vi "Server.vi"() -> ()   [LabVIEW 2020]
uses:
  source/Value/Value/Value.lvclass
  source/Server/Server/Server.lvclass
  source/Server/Source/Source.lvclass
  source/Server/Server.lvlib
  2ff34015-19c1-41a1-a1e8-1eab219b517a.vi
  7054ff5f-c778-4b9f-bf9e-4a55a1cdcc59.vi
  4fabb87d-4e15-4188-883f-208453235fd8.vi
  6c06fff3-e822-4e92-b24f-bdc271668697.vi
  0073a8bc-0586-4490-b945-e374f2b6411c.vi
panel:
  in  "Value":dbl
  in  "Increment":bool
  in  "stop":bool
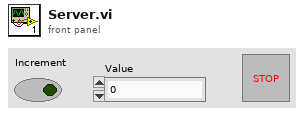
[diagram p1: front panel]
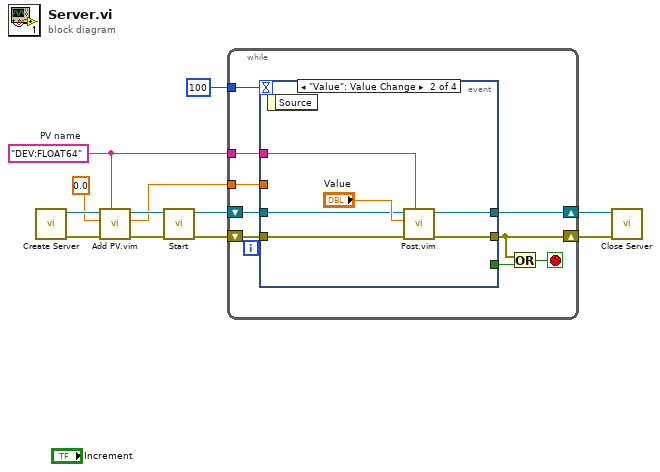
[diagram p0: block diagram]
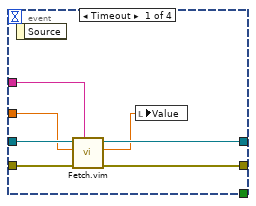
[diagram p2: hidden frame]
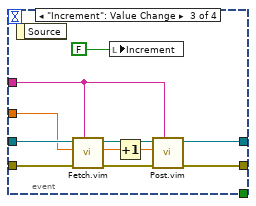
[diagram p3: hidden frame]
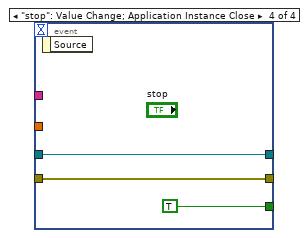
[diagram p4: hidden frame]
diagram:
  w4 = "DEV:FLOAT64"  # PV name
  n1 = call "Create Server.vi"() -> ("error out"=w12:errorcluster, "Server"=w11:refnum<class "Server.lvclass">)  [unwired: 10 in]
  n2 = call "Add PV.vim"("PV name"=w4, "error in"=w12, "initial value"=0.0, "Server in"=w11) -> ("error out"=w7:errorcluster, "value"=w1:dbl, "Server out"=w8:refnum<class "Server.lvclass">)  [unwired: 5 in]
  n3 = call-dynamic "Start.vi"("error in (no error)"=w7, "Server in"=w8) -> ("error out"=w5:errorcluster, "Server out"=w6:refnum<class "Server.lvclass">)  [unwired: 8 in]
  n4 = while {
    tunnel: w4 -> [w20]
    shift-right: [w18] -> w9
    shift-left: w6 -> [w19]
    shift-right: [w15] -> w10
    shift-left: w5 -> [w21]
    tunnel: 100 ("Numeric") -> [w14]
    tunnel: w1 -> [w13]
    stop <- w16 stop-if-true
    n5 = event shown="[1] \"Value\": Value Change" {
      selector: _ -> [_ _ _ _]
      dyn-events: _ -> [_ _ _ _]
      timeout: w14 -> [_ _ _ _]
      tunnel: w21 -> [w27 w34 w45 w47]
      tunnel: w20 -> [w28 w32 w37 _]
      tunnel: w19 -> [w26 w31 w44 w46]
      tunnel: [w24 w29 w35 w47] -> w15
      tunnel: [w25 w30 w36 w46] -> w18
      tunnel: [_ _ _ TRUE] -> w17
      tunnel: w13 -> [w23 _ w41 _]
      event Timeout {
        n6 = event-data() -> ()  [unwired: 1 in, 1 out]
        n7 = call "Fetch.vim"("PV name"=w28, "error in"=w27, "default"=w23, "Server in"=w26) -> ("error out"=w24:errorcluster, "value"=w22:dbl, "Server out"=w25:refnum<class "Server.lvclass">)  [unwired: 5 in]
        n8 = local write "Value"(w22) -> ()
      }
      event "Value": Value Change {
        n9 = event-data() -> ()  [unwired: 1 in, 1 out]
        n10 = call "Post.vim"("PV name"=w32, "error in"=w34, "value in"="Value", "Server in"=w31) -> ("error out"=w29:errorcluster, "Server out"=w30:refnum<class "Server.lvclass">)  [unwired: 5 in, 1 out]
      }
      event "Increment": Value Change {
        n11 = event-data() -> ()  [unwired: 1 in, 1 out]
        n12 = call "Fetch.vim"("PV name"=w37, "error in"=w45, "default"=w41, "Server in"=w44) -> ("error out"=w40:errorcluster, "value"=w42:dbl, "Server out"=w38:refnum<class "Server.lvclass">)  [unwired: 5 in]
        n13 = local write "Increment"(FALSE ("Increment")) -> ()
        n14 = Increment(x=w42) -> (x+1=w39:dbl)
        n15 = call "Post.vim"("PV name"=w37, "error in"=w40, "value in"=w39, "Server in"=w38) -> ("error out"=w35:errorcluster, "Server out"=w36:refnum<class "Server.lvclass">)  [unwired: 5 in, 1 out]
      }
      event "stop": Value Change; Application Instance Close {
        n16 = event-data() -> ()  [unwired: 1 in, 1 out]
      }
    }
    n17 = Or(x=w15, y=w17) -> (x .or. y?=w16:bool)
  }
  n18 = call "Close Server.vi"("error in (no error)"=w10, "Server"=w9) -> ()  [unwired: 9 in, 1 out]
